vi "window function V1.vi"(5 "?":T1 {"I&Q data" format="%.4e"; "sampling freq." format="%.5p"}) -> (0 "window parameters":T2 {"offset" format="%.4p"; "window width" format="%.4p"}, 1 "Offset":i32(slide) scale=1.3706896698527875..4.57758625592346, 2 "width":i32)   [LabVIEW 2022 SP3]
doc: "Graphs the I and Q waveforms. Choose the time window and the offset. The offset determines the width of the time slice in the final spectrogram."
panel:
  out "sampling period":sgl format="%.4p"
  in  "power of 2":u8=8 step=1
  in  "Offset":i32(slide)=50 min=0 max=50000 scale=0.0..256.0
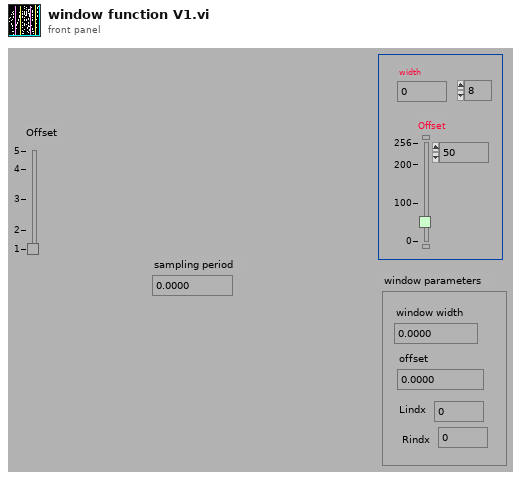
[diagram p1: front panel]
types:
  T1 = cluster{"number of scans":u32, "sampling freq.":sgl, "I&Q data":sgl[][]}
  T2 = cluster{"window width":sgl, "offset":sgl, "Lindx":i32, "Rindx":i32}
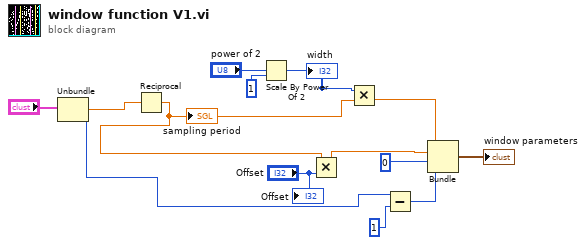
[diagram p0: block diagram]
diagram:
  n1 = Unbundle("?") -> ("number of scans"=w3:u32, "sampling freq."=w13:sgl)  [unwired: 1 out]
  n2 = Reciprocal(x=w13) -> (1/x=w12:sgl)
  "sampling period" <- w12
  n3 = Scale By Power Of 2(n="power of 2", x=1) -> (x*2^n=w6:i32)
  "width" <- w6
  n4 = Multiply(x=w12, y="Offset") -> (x*y=w8:sgl)
  n5 = Multiply(x=w6, y=w12) -> (x*y=w9:sgl)
  n6 = Subtract(x=w3, y=1) -> (x-y=w2:u32)
  n7 = Bundle(w9, w8, 0, w2) -> (→"window parameters":cluster{sgl, sgl, i32, u32})  [unwired: 1 in]
  "Offset" <- "Offset"
